vi "ZLIB Copy Raw File__ogtk.vi"(7 "zip Refnum":T2, 8 "error in (no error)":errorcluster, 10 "name (empty: use current)":string, 11 "unzip Refnum":T1) -> (0 "error out":errorcluster, 3 "unzip Refnum out":T1, 5 "zip Refnum out":T2)   [LabVIEW 2014, in "ZLIB.lvlib"]
doc: "Copies a file in raw mode from an unzip session into a zip session."
uses:
  ZLIB.lvlib
  ZLIB Unzip Handle__ogtk.ctl
  ZLIB Zip Handle__ogtk.ctl
panel:
  # "Please visit http://www.OpenG.org to learn about the\nOpen Source LabVIEW software movement.\n\nNOTICE -- YOU MUST LEAVE THIS NOTICE IN PLACE.  PER THE TERMS OF THE LICENSE BELOW, YOU MAY SUBLICENSE THIS SOFTWARE \nIN ANY WAY THAT DOES NOT CONFLICT WITH THIS LICENSE.\n\n### BSD License (http://www.opensource.org/licenses/bsd-license.php) Begin ###\n \nCopyright (C) 2002-2007 Rolf Kalbermatter rolf.kalbermatter@citeng.com\nCopyright (C) 2002 Jim Kring jim@jimkring.com\n\nAll rights reserved.\n\nRedistribution and use in source and binary forms, with or without modification, are permitted provided that the following conditions are met:\n\n    * Redistributions of source code must retain the above copyright notice, this list of conditions and the following disclaimer.\n    * Redistributions in binary form must reproduce the above copyright notice, this list of conditions and the following disclaimer in the \n       documentation and/or other materials provided with the distribution.\n    * Neither the name of SciWare, James Kring, Inc., nor the names of its contributors may be used to endorse or promote products derived \n       from this software without specific prior written permission.\n\nTHIS SOFTWARE IS PROVIDED BY THE COPYRIGHT HOLDERS AND CONTRIBUTORS \"AS IS\" AND ANY EXPRESS OR IMPLIED WARRANTIES, \nINCLUDING, BUT NOT LIMITED TO, THE IMPLIED WARRANTIES OF MERCHANTABILITY AND FITNESS FOR A PARTICULAR PURPOSE ARE \nDISCLAIMED. IN NO EVENT SHALL THE COPYRIGHT OWNER OR CONTRIBUTORS BE LIABLE FOR ANY DIRECT, INDIRECT, INCIDENTAL,\n SPECIAL, EXEMPLARY, OR CONSEQUENTIAL DAMAGES (INCLUDING, BUT NOT LIMITED TO, PROCUREMENT OF SUBSTITUTE GOODS OR \nSERVICES; LOSS OF USE, DATA, OR PROFITS; OR BUSINESS INTERRUPTION) HOWEVER CAUSED AND ON ANY THEORY OF LIABILITY, \nWHETHER IN CONTRACT, STRICT LIABILITY, OR TORT (INCLUDING NEGLIGENCE OR OTHERWISE) ARISING IN ANY WAY OUT OF THE USE \nOF THIS SOFTWARE, EVEN IF ADVISED OF THE POSSIBILITY OF SUCH DAMAGE.\n\n### BSD License End ###"
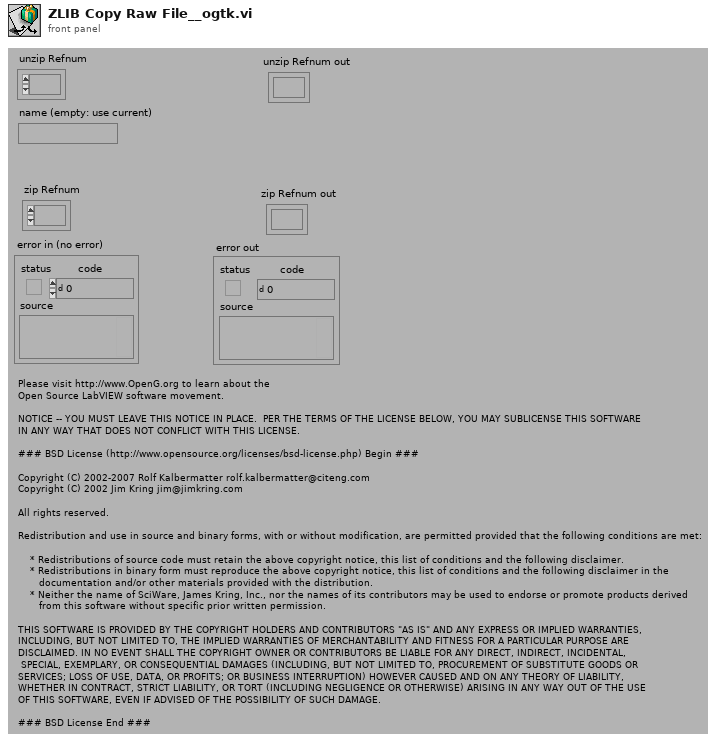
[diagram p1: front panel]
types:
  T1 = typedef "ZLIB.lvlib/ZLIB Unzip Handle__ogtk.ctl" = refnum<k1>
  T2 = typedef "ZLIB.lvlib/ZLIB Zip Handle__ogtk.ctl" = refnum<k1>
  T3 = typedef "ZLIB.lvlib/ZLIB File Info__ogtk.ctl" = cluster{"version":u32, "version needed":u32, "encrypted":bool, "flag":u32, "compression":i32, "dos date":u32, "crc":u32, "compressed size":u32, "uncompressed size":u32, "extra info":string, "file comment":string, "disk num start":u32, "internal fa":u32, "external fa":u32, "file timestamp":u32}
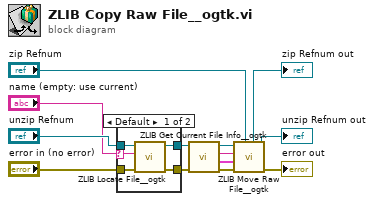
[diagram p0: block diagram]
diagram:
  n1 = case shown="Default" "name (empty: use current)" {
    selector: "name (empty: use current)" -> [w14 _]
    tunnel: [w18 w20] -> w9
    tunnel: [w17 w19] -> w8
    tunnel: "unzip Refnum" -> [w16 w20]
    tunnel: "error in (no error)" -> [w15 w19]
    frame Default {
      n2 = call "ZLIB Locate File__ogtk.vi"("error in (no error)"=w15, "name (empty: -)"=w14, "unzip Refnum"=w16) -> ("error out"=w17:errorcluster, "unzip Refnum out"=w18:T1)  [unwired: 3 in]
    }
    frame "" {
    }
  }
  n3 = call "ZLIB Get Current File Info__ogtk.vi"("error in (no error)"=w8, "unzip Refnum"=w9) -> ("error out"=w5:errorcluster, "file info"=w1:T3, "name"=w3:string, "unzip Refnum out"=w6:T1)  [unwired: 6 in]
  n4 = call "ZLIB Move Raw File__ogtk.vi"("zip Refnum"="zip Refnum", "error in (no error)"=w5, "file info"=w1, "name"=w3, "unzip Refnum"=w6) -> ("error out"=→"error out":errorcluster, "unzip Refnum out"=→"unzip Refnum out":T1, "zip Refnum out"=→"zip Refnum out":T2)  [unwired: 4 in]
